vi "SEA 9811_SoftwareManual.vi"   [LabVIEW 2017]
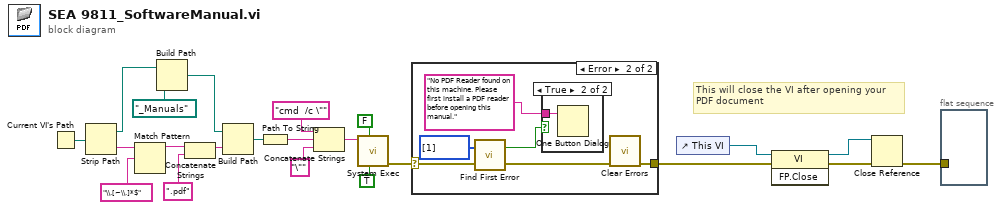
[diagram p0: block diagram]
diagram:
  # "This will close the VI after opening your\nPDF document"
  n1 = Current VI's Path() -> (path=w11:path)
  n2 = Strip Path(path=w11) -> (stripped path=w2:path, name=w10:string)
  n3 = Match Pattern(string=w10, regular expression="\\.[~\\.]*$") -> (before substring=w8:string)  [unwired: 4 out]
  n4 = Build Path(base path=w2, name or relative path=path "_Manuals") -> (appended path=w1:path)
  n5 = Concatenate Strings(w8, ".pdf" ("substring (\"\")")) -> (w6:string)
  n6 = Build Path(base path=w1, name or relative path=w6) -> (appended path=w5:path)
  n7 = Path To String(path=w5) -> (string=w17:string)
  n8 = Concatenate Strings("cmd  /c \"", w17, "\"") -> (w15:string)
  n9 = call <vilib>:"System Exec.vi"("run minimized? (F)"=TRUE, "wait until completion? (T)"=FALSE, "command line"=w15) -> ("error out"=w12:errorcluster)  [unwired: 3 in, 5 out]
  n10 = case shown="Error" w12 {
    selector: w12 -> [w23 w29]
    tunnel: [w23 w26] -> w19
    frame No Error {
    }
    frame Error {
      n11 = call <vilib>:"Find First Error.vi"("error in (no error)"=w29, "error codes"=i32[] [1]) -> ("error out"=w27:errorcluster, "error?"=w25:bool)  [unwired: 2 in]
      n12 = case shown="True" w25 {
        tunnel: "No PDF Reader found on this machine. Please first install a PDF reader before opening this manual." -> [_ w30]
        frame False {
        }
        frame True {
          n13 = One Button Dialog(message=w30) -> ()  [unwired: 1 in, 1 out]
        }
      }
      n14 = call <vilib>:"Clear Errors.vi"("error in (no error)"=w27) -> ("error out"=w26:errorcluster)  [unwired: 5 in, 1 out]
    }
  }
  n15 = control-ref of="This VI"() -> (w20:refnum<vi>)
  n16 = invoke class="VI" method="FP.Close"(reference=w20, error in=w19) -> (reference out=w22:refnum<vi>, error out=w21:errorcluster)  [unwired: 1 in, 1 out]
  n17 = Close Reference(reference=w22, error in (no error)=w21) -> (error out=w4:errorcluster)
  n18 = flat-sequence {
    tunnel: w4 -> [_]
    frame #0 {
    }
  }
